vi "Read Chapter Infos.vi"(0 "PDF Report IN":refnum<class "PDF Report Class.lvclass">, 2 "Type and run direction":T1=enum."ASCII", 5 "Chapter":refnum<k24>, 7 "Section":refnum<k24>, 9 "Y before":sgl, 11 "error in (no error)":errorcluster, 13 "Title":string) -> (4 "PDF Report OUT":refnum<class "PDF Report Class.lvclass">, 15 "error out":errorcluster)   [LabVIEW 2020, in "Exaprom PDF.lvlib"]
doc: "Version 1.1\nDeveloped by Jean-Marc Simard\nCopyright © 2012, Exaprom Inc.\nAll rights reserved.\nLicense: BSD\n\nWith iTextSharp 4.1.6 (http://itextsharp.sourceforge.net)\nunder Mozilla Public License Version 1.1\n(http://www.mozilla.org/MPL/MPL-1.1.html)"
uses:
  <userlib>/labview-PDF-writer-master/Exaprom PDF.lvlib
  <userlib>/labview-PDF-writer-master/LV Class/PDF Report Class/PDF Report Class.lvclass
  C:/Program Files (x86)/National Instruments/LabVIEW 2020/user.lib/labview-PDF-writer-master/DLL/itextsharp.dll
  DLL/itextsharp.dll
  <userlib>/labview-PDF-writer-master/Controls/Text Controls/Unicode/Type and run direction.ctl
  <userlib>/labview-PDF-writer-master/Controls/Chapter Controls/TOC Line.ctl
panel:
  out "Content 2":string
  out "Content":string
  # "类型和运行方向"
  # "根据编码类型 调整方向"
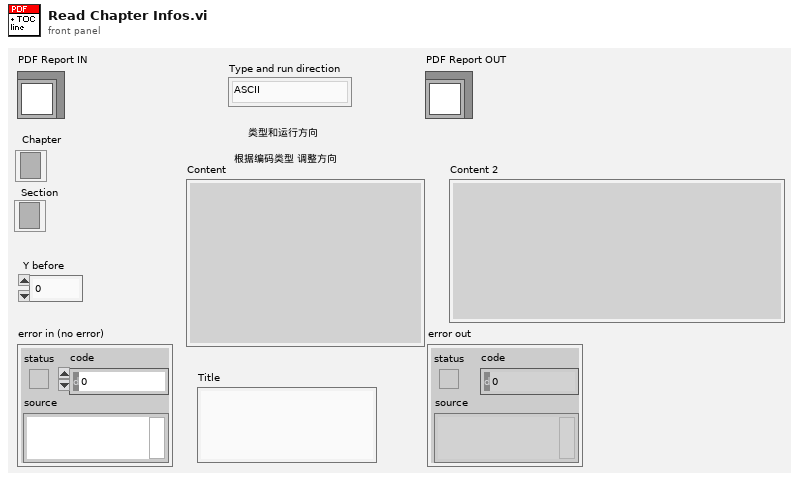
[diagram p1: front panel]
types:
  T1 = typedef "Exaprom PDF.lvlib/Type and run direction.ctl" = enum16{"Select", "ASCII", "UTF-16", "UTF-16 (default)", "UTF-16 (LTR)", "UTF-16 (RTL)"}
  T2 = typedef "Exaprom PDF.lvlib/TOC Line.ctl" = cluster{"Title":string, "Level":u16, "GoTo Page":u16, "GoTo Position":u16, "Destination":string, "Type & run direction":T1}
  T3 = typedef "Exaprom PDF.lvlib/Page dimensions.ctl" = cluster{"Start at page":i32, "Page Size":T4, "Orientation":T5, "widht":sgl, "height":sgl, "Margin left":sgl, "Margin right":sgl, "Margin top":sgl, "Margin bottom":sgl, "X0":sgl, "X1":sgl, "Y0":sgl, "Y1":sgl}
  T4 = typedef "Exaprom PDF.lvlib/Page size.ctl" = i32
  T5 = typedef "Exaprom PDF.lvlib/Page Orientation.ctl" = enum16{"Portrait", "Landscape"}
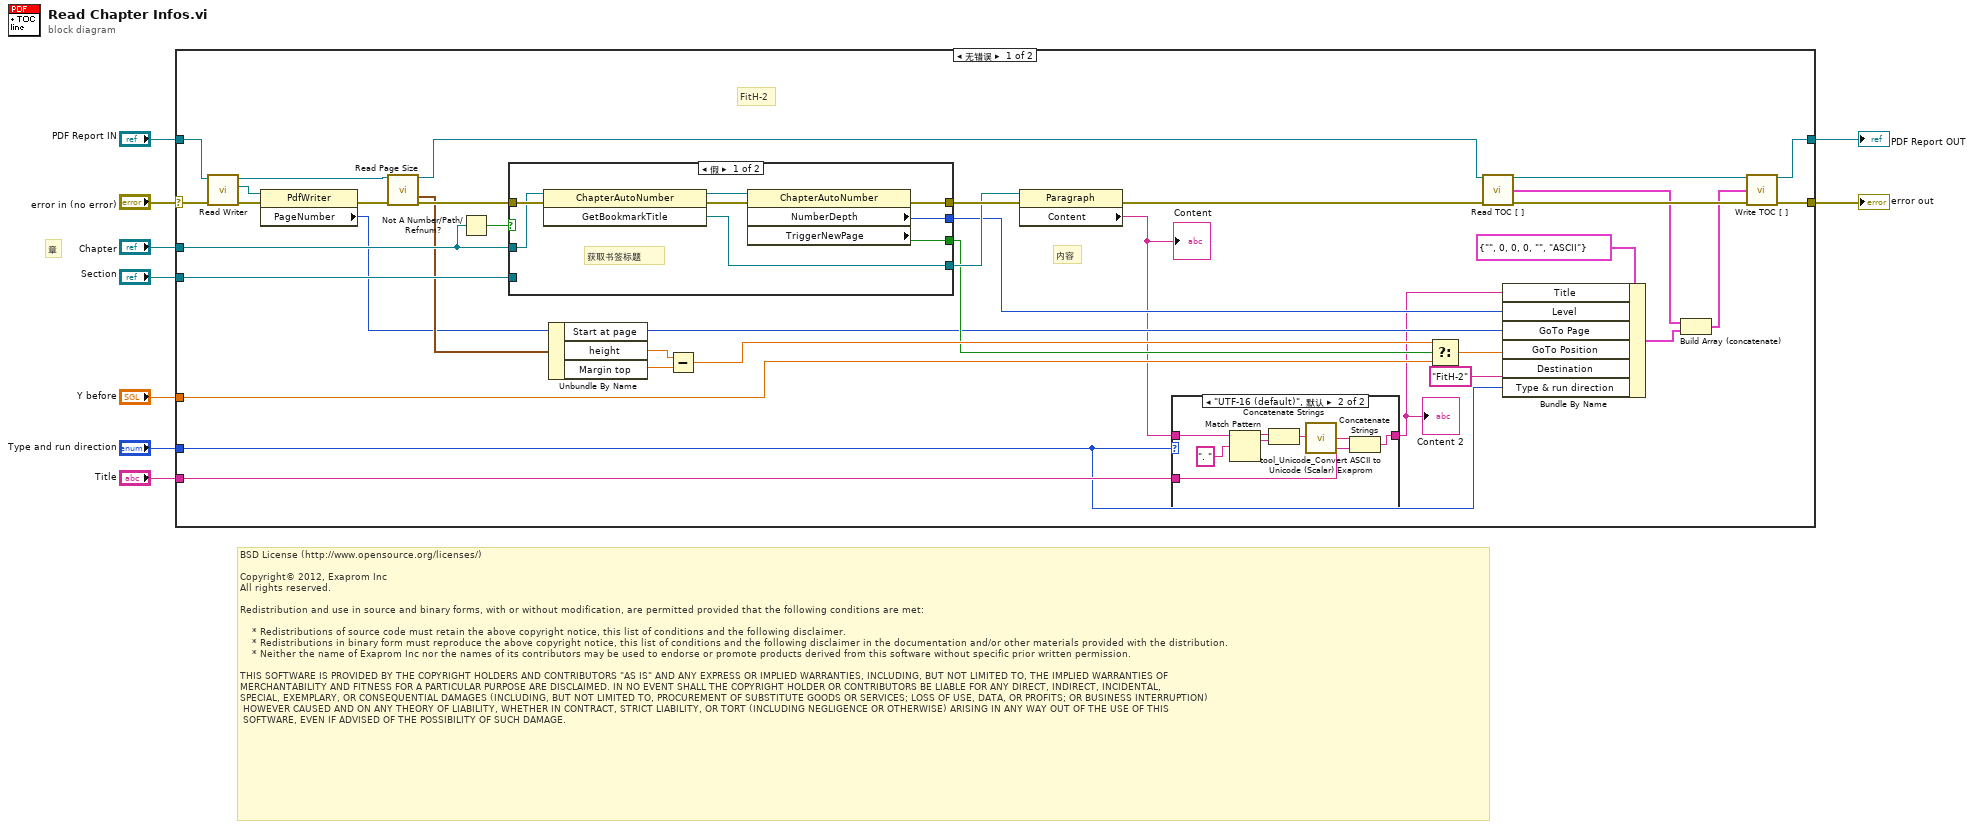
[diagram p0: block diagram]
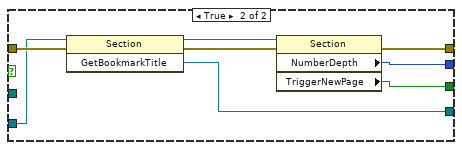
[diagram p3: hidden frame]
diagram:
  # "章"
  # "BSD License (http://www.opensource.org/licenses/)\n\nCopyright© 2012, Exaprom Inc\nAll rights reserved.\n\nRedistribution and use in source and binary forms, with or without modification, are permitted provided that the following conditions are met:\n\n    * Redistributions of source code must retain the above copyright notice, this list of conditions and the following disclaimer.\n    * Redistributions in binary form must reproduce the above copyright notice, this list of conditions and the following disclaimer in the documentation and/or other materials provided with the distribution.\n    * Neither the name of Exaprom Inc nor the names of its contributors may be used to endorse or promote products derived from this software without specific prior written permission.\n\nTHIS SOFTWARE IS PROVIDED BY THE COPYRIGHT HOLDERS AND CONTRIBUTORS \"AS IS\" AND ANY EXPRESS OR IMPLIED WARRANTIES, INCLUDING, BUT NOT LIMITED TO, THE IMPLIED WARRANTIES OF \nMERCHANTABILITY AND FITNESS FOR A PARTICULAR PURPOSE ARE DISCLAIMED. IN NO EVENT SHALL THE COPYRIGHT HOLDER OR CONTRIBUTORS BE LIABLE FOR ANY DIRECT, INDIRECT, INCIDENTAL,\nSPECIAL, EXEMPLARY, OR CONSEQUENTIAL DAMAGES (INCLUDING, BUT NOT LIMITED TO, PROCUREMENT OF SUBSTITUTE GOODS OR SERVICES; LOSS OF USE, DATA, OR PROFITS; OR BUSINESS INTERRUPTION)\n HOWEVER CAUSED AND ON ANY THEORY OF LIABILITY, WHETHER IN CONTRACT, STRICT LIABILITY, OR TORT (INCLUDING NEGLIGENCE OR OTHERWISE) ARISING IN ANY WAY OUT OF THE USE OF THIS\n SOFTWARE, EVEN IF ADVISED OF THE POSSIBILITY OF SUCH DAMAGE."
  n1 = case shown="无错误" "error in (no error)" {
    selector: "error in (no error)" -> [w38 w72]
    tunnel: "PDF Report IN" -> [w16 w71]
    tunnel: [w20 w71] -> w8
    tunnel: [w23 w72] -> w7
    tunnel: "Chapter" -> [w44 _]
    tunnel: "Section" -> [w43 _]
    tunnel: "Y before" -> [w31 _]
    tunnel: "Title" -> [w13 _]
    tunnel: "Type and run direction" -> [w10 _]
    frame No Error {
      # "内容"
      # "FitH-2"
      n2 = call-dynamic "Read Writer.vi"("error in (no error)"=w38, "PDF Report Class in"=w16) -> ("error out"=w18:errorcluster, "Writer"=w19:refnum<k24>, "PDF Report Class out"=w15:refnum<class "PDF Report Class.lvclass">)  [unwired: 7 in]
      n3 = property class="PdfWriter"(reference=w19, error in=w18) -> (error out=w17:errorcluster, "PageNumber"=w14:i32)  [unwired: 1 out]
      n4 = call <userlib>:"Read Page Size.vi"("PDF Report"=w15, "error in (no error)"=w17) -> ("PDF Report duplicate"=w26:refnum<class "PDF Report Class.lvclass">, "Page (points)"=w36:T3, "error out"=w37:errorcluster)  [unwired: 10 in, 1 out]
      n5 = Not A Number/Path/Refnum?(number/path/refnum=w44) -> (NaN/Path/Refnum?=w45:bool)
      n6 = case shown="假" w45 {
        tunnel: w37 -> [w62 w70]
        tunnel: w44 -> [w60 _]
        tunnel: w43 -> [_ w67]
        tunnel: [w58 w66] -> w39
        tunnel: [w57 w65] -> w32
        tunnel: [w56 w64] -> w41
        tunnel: [w55 w63] -> w42
        frame False {
          # "获取书签标题"
          n7 = invoke class="ChapterAutoNumber" method="GetBookmarkTitle"(reference=w60, error in=w62) -> (reference out=w61:refnum<k24>, error out=w59:errorcluster, "GetBookmarkTitle"=w56:refnum<k24>)  [unwired: 1 in]
          n8 = property class="ChapterAutoNumber"(reference=w61, error in=w59) -> (error out=w55:errorcluster, "NumberDepth"=w58:i32, "TriggerNewPage"=w57:bool)  [unwired: 1 out]
        }
        frame True {
          n9 = invoke class="Section" method="GetBookmarkTitle"(reference=w67, error in=w70) -> (reference out=w69:refnum<k24>, error out=w68:errorcluster, "GetBookmarkTitle"=w64:refnum<k24>)  [unwired: 1 in]
          n10 = property class="Section"(reference=w69, error in=w68) -> (error out=w63:errorcluster, "NumberDepth"=w66:i32, "TriggerNewPage"=w65:bool)  [unwired: 1 out]
        }
      }
      n11 = Unbundle By Name(w36) -> ("height"=w35:sgl, "Margin top"=w34:sgl)  [unwired: 1 out]
      n12 = Subtract(x=w35, y=w34) -> (x-y=w33:sgl)
      n13 = property class="Paragraph"(reference=w41, error in=w42) -> (error out=w28:errorcluster, "Content"=w12:string)  [unwired: 1 out]
      "Content" <- w12
      n14 = case shown="\"UTF-16 (default)\", 默认" w10 {
        tunnel: w12 -> [w46 w54]
        tunnel: w13 -> [_ w48]
        tunnel: [w46 w47] -> w11
        frame "ASCII" {
        }
        frame "UTF-16 (default)", Default {
          n15 = Match Pattern(string=w54, regular expression=". ") -> (before substring=w52:string, match substring=w51:string)  [unwired: 1 in, 2 out]
          n16 = Concatenate Strings(w52, w51) -> (w50:string)
          n17 = call <userlib>:"tool_Unicode_Convert ASCII to Unicode (Scalar) Exaprom.vi"("ASCII"=w50) -> ("Unicode"=w49:string)  [unwired: 4 in]
          n18 = Concatenate Strings(w49, w48) -> (w47:string)
        }
      }
      "Content 2" <- w11
      n19 = Select(t=w33, s=w32, f=w31) -> (s? t:f=w30:sgl)
      n20 = call-dynamic "Read TOC [ ].vi"("PDF Report Class in"=w26, "error in (no error)"=w28) -> ("PDF Report Class out"=w21:refnum<class "PDF Report Class.lvclass">, "TOC [ ]"=w25:T2[], "error out"=w27:errorcluster)  [unwired: 11 in]
      n21 = Bundle By Name(cluster=T2 {"Title"="", "Level"=0, "GoTo Page"=0, "GoTo Position"=0, "Destination"="", "Type & run direction"=enum."ASCII"} ("TOC Line"), "Title"=w11, "Level"=w39, "GoTo Page"=w14, "GoTo Position"=w30, "Destination"="FitH-2", "Type & run direction"=w10) -> (w24:T2)
      n22 = Build Array (concatenate)(w25, w24) -> (w22:T2[])
      n23 = call-dynamic "Write TOC [ ].vi"("PDF Report Class in"=w21, "TOC [ ]"=w22, "error in (no error)"=w27) -> ("PDF Report Class out"=w20:refnum<class "PDF Report Class.lvclass">, "error out"=w23:errorcluster)  [unwired: 11 in]
    }
    frame Error {
    }
  }
  "PDF Report OUT" <- w8
  "error out" <- w7
